vi "Asana Authentication.vi"(8 "error in (no error)":errorcluster, 9 "Authentication Info":T1={"Client ID"="", "Client Secret"="", "Redirect URI"="", "Token Endpoint"="https://app.asana.com/-/oauth_token", "Scope"=""}, 10 "Refresh Token In":string) -> (0 "error out":errorcluster, 1 "Authentication Header":T2[](array[typedef]), 2 "Refresh Token Out":string, 3 "Timeout":dbl)   [LabVIEW 2016]
uses:
  <vilib>/addons/_JKI.lib/REST Client/classes/REST Client/HTTP Header.ctl
  OAuth/OO OAuth/scope_needed.ctl
  <vilib>/addons/_JKI.lib/REST Client/classes/REST Client/REST Client.lvclass
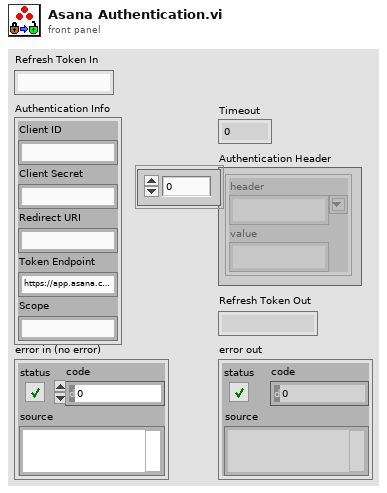
[diagram p1: front panel]
types:
  T1 = cluster{"Client ID":string, "Client Secret":string, "Redirect URI":string, "Token Endpoint":string, "Scope":string}
  T2 = typedef "REST Client.lvlib/REST Client.lvclass/HTTP Header.ctl" = cluster{"header":string, "value":string}
  T3 = typedef "scope_needed.ctl" = enum16{"No", "Yes"}
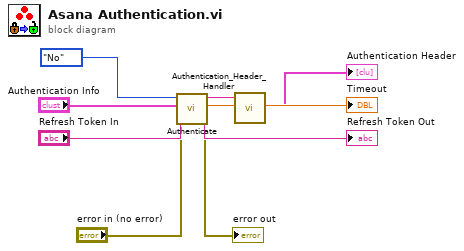
[diagram p0: block diagram]
diagram:
  n1 = call "Authenticate.vi"("error in (no error)"="error in (no error)", "Refresh Token"="Refresh Token In", "Authentication Info"="Authentication Info", "Scope Needed?"=scope_needed."No") -> ("error out"=→"error out":errorcluster, "Refresh Token"=→"Refresh Token Out":string, "Timeout"=→"Timeout":dbl, "Access Token"=w9:string)  [unwired: 4 in]
  n2 = call "Authentication_Header_Handler.vi"("String"=w9) -> ("output array"=→"Authentication Header":T2[])  [unwired: 10 in]
